vi "信号输出使能.vi"(0 "VISA资源名称":refnum<visa-resource-name>, 7 "信号输出":bool, 11 "错误输入（无错误）":errorcluster) -> (4 "元素 2":string, 15 "错误输出 2":errorcluster caption="错误输出")   [LabVIEW 2014]
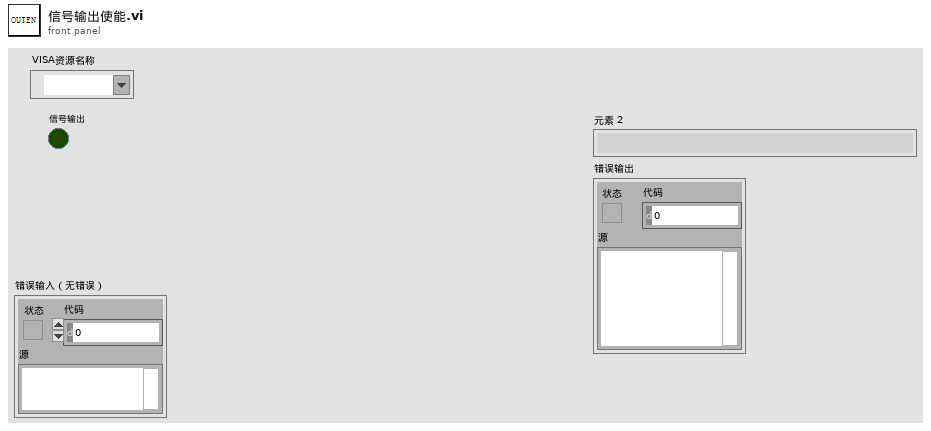
[diagram p1: front panel]
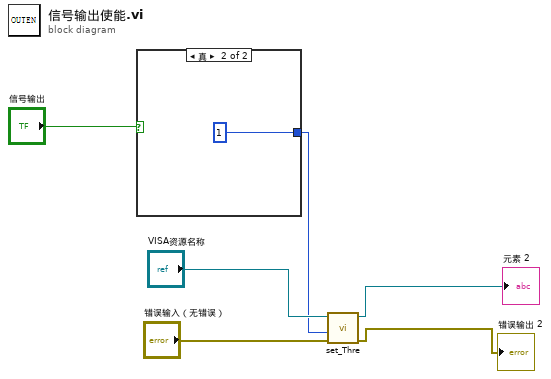
[diagram p0: block diagram]
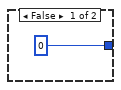
[diagram p2: hidden frame]
diagram:
  n1 = case shown="真" "信号输出" {
    tunnel: [0 1] -> w2
    frame False {
    }
    frame True {
    }
  }
  n2 = call "set_Thre.vi"("错误输入（无错误）"="错误输入（无错误）", "命令"=w2, "VISA资源名称"="VISA资源名称") -> ("错误输出"=→"错误输出 2":errorcluster, "VISA资源名称输出"=→"元素 2":refnum<visa-resource-name>)  [unwired: 7 in]
